vi "ConvertStrToInt.vi"(11 "string":string) -> (3 "result":i32)   [LabVIEW 2018, in "Library-DataConvert.lvlib"]
uses:
  Library-DataConvert.lvlib
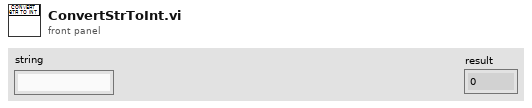
[diagram p1: front panel]
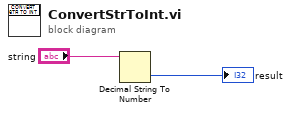
[diagram p0: block diagram]
diagram:
  n1 = Decimal String To Number(string="string") -> (number=→"result":i32)  [unwired: 2 in, 1 out]
